vi "GetAxisInfoEx.vi"(0 "axis in":cluster{"keyHandle":u32, "nodeId":u16}={"keyHandle"=0, "nodeId"=1}, 11 "error in (no error)":errorcluster) -> (4 "axis out":cluster{"keyHandle":u32, "nodeId":u16}={"keyHandle"=0, "nodeId"=1}, 6 "axis state":T2(ring), 8 "targetReached":i32, 10 "axis data ex":T1, 15 "error out":errorcluster)   [LabVIEW 2019, in "maxonEPOS.lvlib"]
doc: "<B>GetAxisInfos</B> reads the actual position, velocity and current from the device and looks if the target is reached."
uses:
  Examples/maxonEPOS.lvlib
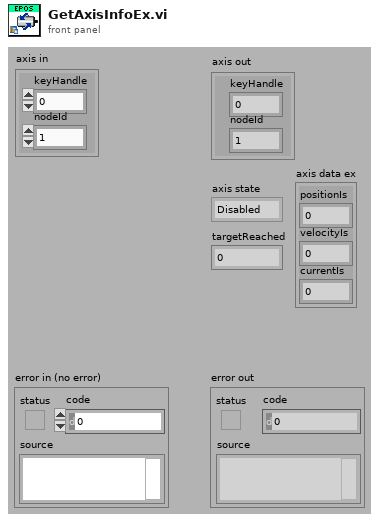
[diagram p1: front panel]
types:
  T1 = cluster{"positionIs":i32, "velocityIs":i32, "currentIs":i32}
  T2 = enum16{"Disabled", "Enabled", "Quickstop", "Fault"}
  T3 = cluster{"positionIs":i32, "velocityIs":i32, "currentIs":i16}
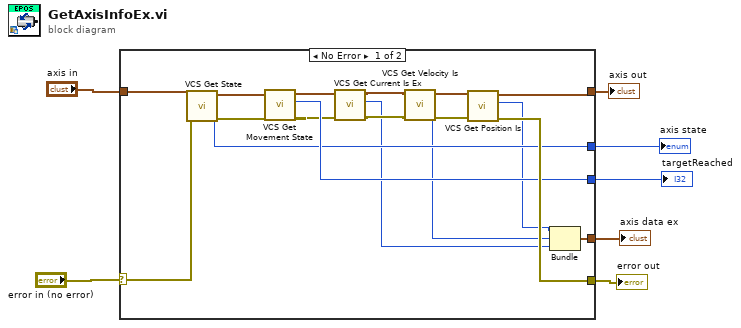
[diagram p0: block diagram]
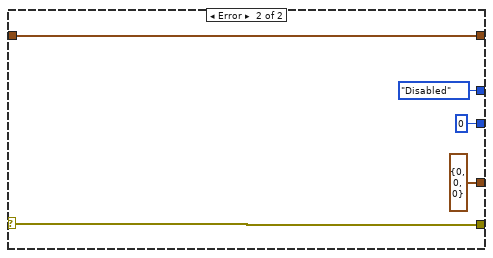
[diagram p2: hidden frame]
diagram:
  n1 = case shown="No Error" "error in (no error)" {
    selector: "error in (no error)" -> [w19 w30]
    tunnel: [w23 w30] -> w6
    tunnel: [w24 w29] -> w5
    tunnel: "axis in" -> [w20 w29]
    tunnel: [w21 0 ("targetReached")] -> w3
    tunnel: [w16 T2."Disabled" ("state")] -> w2
    tunnel: [w13 T3 {"positionIs"=0, "velocityIs"=0, "currentIs"=0}] -> w1
    frame No Error {
      n2 = call "VCS Get State.vi"("error in (no error)"=w19, "axis in"=w20) -> ("error out"=w17:errorcluster, "state"=w16:T2, "axis out"=w18:cluster{"keyHandle":u32, "nodeId":u16})  [unwired: 7 in]
      n3 = call "VCS Get Movement State.vi"("error in (no error)"=w17, "axis in"=w18) -> ("error out"=w9:errorcluster, "targetReached"=w21:i32, "axis out"=w10:cluster{"keyHandle":u32, "nodeId":u16})  [unwired: 7 in]
      n4 = call "VCS Get Current Is Ex.vi"("error in (no error)"=w9, "axis in"=w10) -> ("error out"=w12:errorcluster, "currentIs"=w8:i32, "axis out"=w11:cluster{"keyHandle":u32, "nodeId":u16})  [unwired: 7 in]
      n5 = call "VCS Get Velocity Is.vi"("error in (no error)"=w12, "axis in"=w11) -> ("error out"=w22:errorcluster, "velocityIs"=w14:i32, "axis out"=w25:cluster{"keyHandle":u32, "nodeId":u16})  [unwired: 7 in]
      n6 = call "VCS Get Position Is.vi"("error in (no error)"=w22, "axis in"=w25) -> ("error out"=w23:errorcluster, "positionIs"=w15:i32, "axis out"=w24:cluster{"keyHandle":u32, "nodeId":u16})  [unwired: 7 in]
      n7 = Bundle("positionIs"=w15, "velocityIs"=w14, "currentIs"=w8) -> (w13:T1)  [unwired: 1 in]
    }
    frame Error {
    }
  }
  "error out" <- w6
  "axis out" <- w5
  "targetReached" <- w3
  "axis state" <- w2
  "axis data ex" <- w1
